vi "Keithley Hangar.vi"() -> ()   [LabVIEW 2013]
uses:
  <vilib>/Platform/TimedLoop/XDataNode/timing_clust.ctl
  <vilib>/Platform/TimedLoop/XDataNode/nitl_modes.ctl
  <vilib>/Platform/TimedLoop/XDataNode/wakeup.ctl
  <vilib>/Instr/_visa.llb/VISA Configure Serial Port (Instr).vi
  <vilib>/Platform/TimedLoop/XDataNode/XDataNode.xnode
  <vilib>/Platform/TimedLoop/XDataNode/XDNodeRunTimeDep.lvlib
panel:
  in  "OK Button":bool
  out "read buffer 3":string
  in  "Unit":string(combo)
  in  "Current":dbl
  in  "CUSTOM COMMAND":string(combo)
  in  "stop":bool
  out "error out":errorcluster
  out "read buffer 2":string
  out "Bytes at Port 3":u32
  in  "RUN Keithley Measurement":bool
  in  "flow control (0:none)":u16(ring) items=["None", "XON/XOFF", "RTS/CTS", "XON/XOFF & RTS/CTS", "DTR/DSR", "XON/XOFF & DTR/DSR"]
  in  "stop bits (10: 1 bit)":u16(ring)=10 items=["1.0"=10, "1.5"=15, "2.0"=20]
  in  "parity (0:none)":enum16{"None", "Odd", "Even", "Mark", "Space"}(ring)
  in  "data bits (8)":u16=8 min=5 max=8 step=1
  in  "baud rate (9600)":u32=9600
  in  "VISA resource name":refnum<visa-resource-name>="COM1"
  in  "Keithley delay (ms)":u32=500
  in  "Set Output Current":bool
  out "actual value":string
  out "Bytes at Port":u32
  out "command to Keithley":string
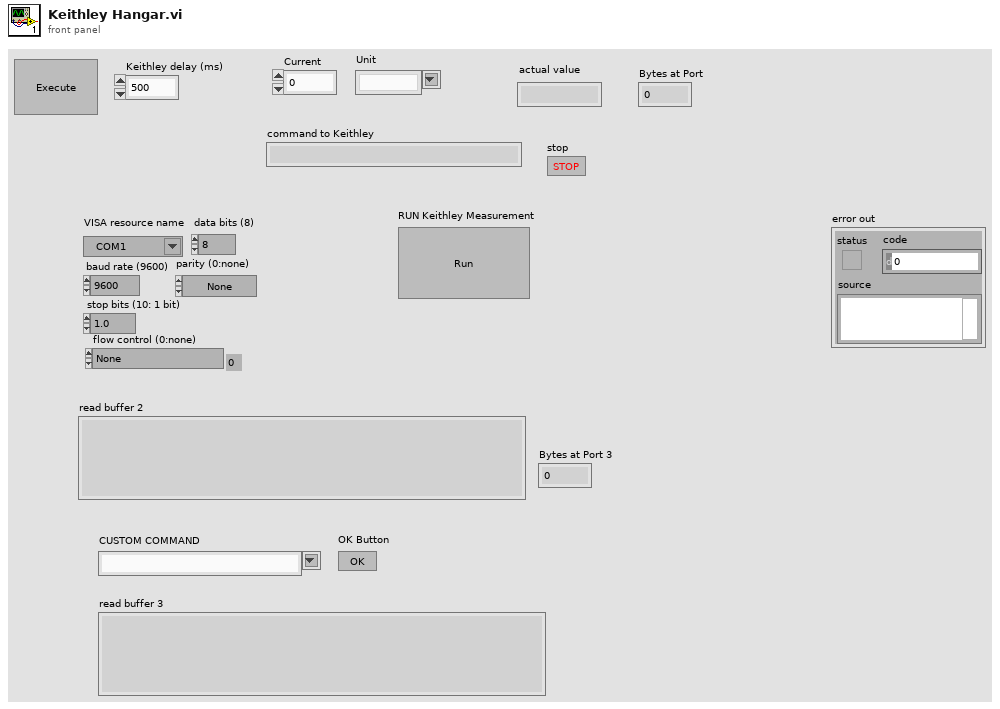
[diagram p1: front panel]
types:
  T1 = typedef "XDNodeRunTimeDep.lvlib/timing_clust.ctl" = cluster{"Expected End [f-1]":u64, "Actual End [f-1]":u64, "Finished Late? [f-1]":bool, "Expected End [i-1]":u64, "Actual End [i-1]":u64, "Finished Late? [i-1]":bool, "Expected Start [i]":u64, "Actual Start [i]":u64, "Expected Start [f]":u64, "Actual Start [f]":u64, "Source Name":string, "Structure Name":string, "Period":i64, "Deadline":i64, "Offset":i64, "Start":i64, "Priority":i32, "Timeout":i32, "Mode":T2, "Wakeup Reason":T3, "Error":errorcluster, "Source Type":string, "Secondary Source Type":string, "Global End Time":u64, "Global Start Time":u64, "Frame Duration":u64, "Iteration Duration":u64, "Assigned CPU":i32, "I/O Scan Engine Mode":u32}
  T2 = typedef "XDNodeRunTimeDep.lvlib/nitl_modes.ctl" = enum32{"No Change", "Process missed periods, maintain original phase", "Discard missed periods, maintain original phase", "Process missed periods, ignore original phase", "Discard missed periods, ignore original phase"}
  T3 = typedef "XDNodeRunTimeDep.lvlib/wakeup.ctl" = enum32{"Normal", "Aborted", "Asynchronous wakeup", "Timing source error", "Timed loop error", "Timeout"}
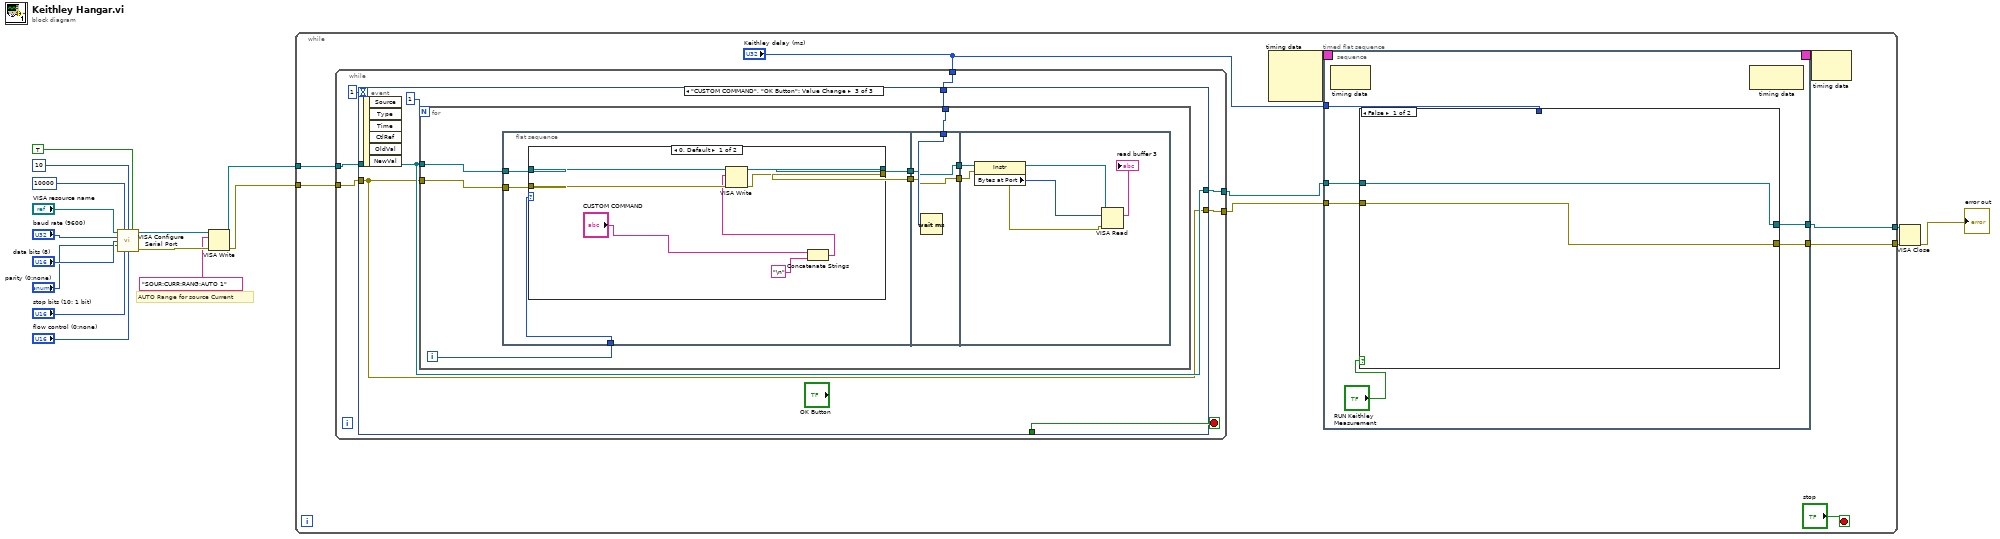
[diagram p0: block diagram]
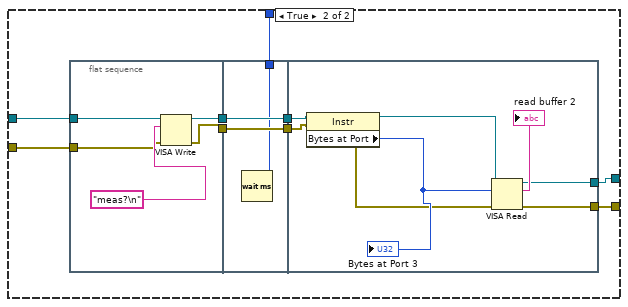
[diagram p2: hidden frame]
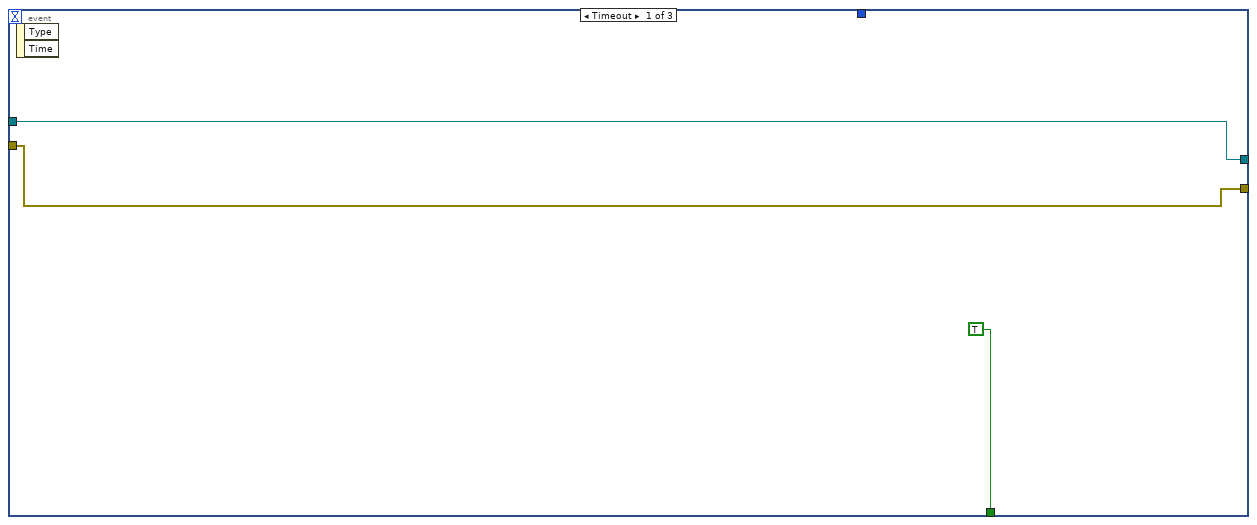
[diagram p3: hidden frame]
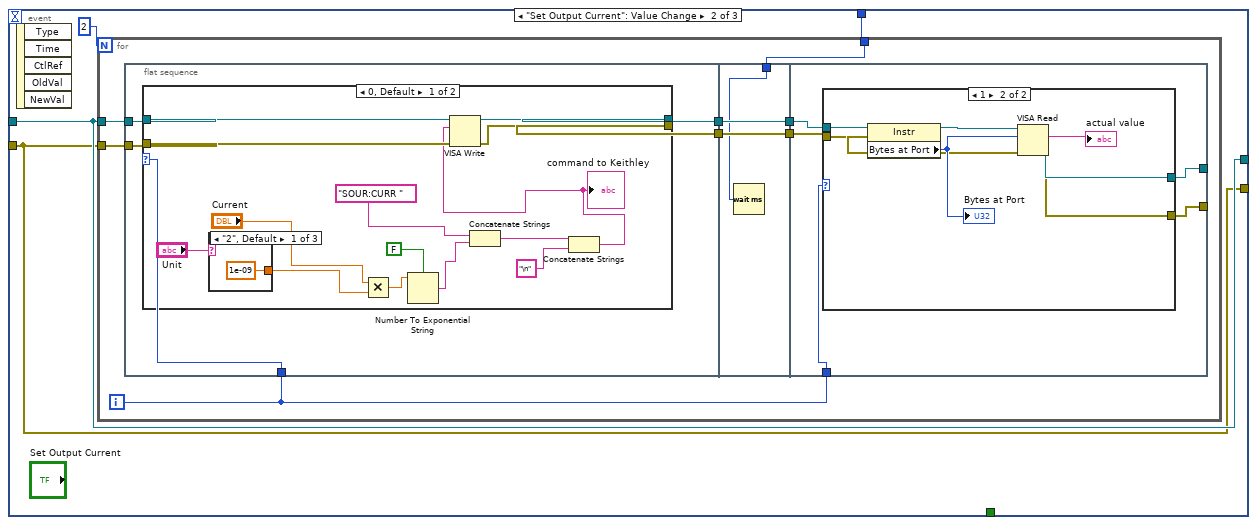
[diagram p4: hidden frame]
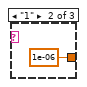
[diagram p5: hidden frame]
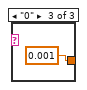
[diagram p6: hidden frame]
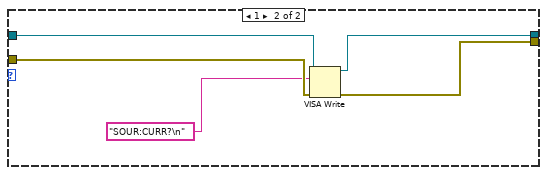
[diagram p7: hidden frame]
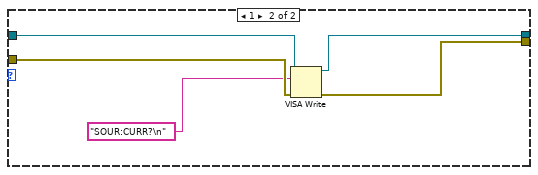
[diagram p9: hidden frame]
diagram:
  # "AUTO Range for source Current"
  n1 = call-poly "VISA Configure Serial Port"("VISA resource name"="VISA resource name", "timeout (10sec)"=u32 10000, "termination char\n(0xA = '\\n' = LF)"=u8 10 ("termination char\n(0xA = '\\n' = LF)"), "Enable Termination\nChar (T)"=TRUE ("Enable Termination\nChar (T)"), "baud rate (9600)"="baud rate (9600)", "data bits (8)"="data bits (8)", "parity (0:none)"="parity (0:none)", "stop bits (10: 1 bit)"="stop bits (10: 1 bit)", "flow control (0:none)"="flow control (0:none)") -> ("VISA resource name out"=w5:refnum<visa-resource-name>, "error out"=w3:errorcluster)  [unwired: 5 in]
  n2 = VISA Write(VISA resource name=w5, write buffer="SOUR:CURR:RANG:AUTO 1", error in (no error)=w3) -> (VISA resource name out=w4:refnum<visa-resource-name>, error out=w2:errorcluster)  [unwired: 1 out]
  n3 = while {
    tunnel: [w25] -> w7
    tunnel: [w24] -> w6
    tunnel: w4 -> [w21]
    tunnel: w2 -> [w20]
    stop <- "stop" stop-if-true
    n4 = while {
      tunnel: "Keithley delay (ms)" -> [w76]
      tunnel: w21 -> [w75]
      tunnel: w20 -> [w74]
      tunnel: [w71] -> w23
      tunnel: [w70] -> w22
      stop <- w72 stop-if-true
      n5 = event shown="[2] \"CUSTOM COMMAND\", \"OK Button\": Value Change" {
        selector: _ -> [_ _ _]
        dyn-events: _ -> [_ _ _]
        timeout: 1 -> [_ _ _]
        tunnel: w76 -> [_ w82 w139]
        tunnel: w75 -> [w78 w81 w138]
        tunnel: w74 -> [w77 w80 w137]
        tunnel: [TRUE _ _] -> w72
        tunnel: [w78 w81 w138] -> w71
        tunnel: [w77 w80 w137] -> w70
        event Timeout {
          n6 = event-data() -> ()  [unwired: 1 in, 2 out]
        }
        event "Set Output Current": Value Change {
          n7 = event-data() -> ()  [unwired: 1 in, 5 out]
          n8 = for {
            N: 2 -> [_]
            tunnel: w82 -> [w86]
            tunnel: w81 -> [w85]
            tunnel: w80 -> [w84]
            i -> [w89]
            n9 = flat-sequence {
              tunnel: [w96] -> w91
              tunnel: w89 -> [w95]
              tunnel: [w94] -> w88
              tunnel: w85 -> [w93]
              tunnel: w84 -> [w92]
              tunnel: w91 -> [w121]
              tunnel: [w121] -> w90
              tunnel: w88 -> [w120]
              tunnel: [w120] -> w87
              tunnel: w86 -> [w119]
              tunnel: w90 -> [w126]
              tunnel: w89 -> [w125]
              tunnel: w87 -> [w124]
              tunnel: [w123] -> _
              tunnel: [w122] -> _
              frame #0 {
                n10 = case shown="0, Default" w95 {
                  tunnel: [w110 w115] -> w96
                  tunnel: [w109 w114] -> w94
                  tunnel: w93 -> [w108 w117]
                  tunnel: w92 -> [w107 w118]
                  frame 0, Default {
                    n11 = case shown="\"2\", Default" "Unit" {
                      tunnel: [1e-09 ("y") 1e-06 ("y") 0.001 ("y")] -> w97
                      frame "2", Default {
                      }
                      frame "1" {
                      }
                      frame "0" {
                      }
                    }
                    n12 = Multiply(x="Current", y=w97) -> (x*y=w100:dbl)
                    n13 = Number To Exponential String(number=w100, 1:FALSE ("use system decimal point (T)")) -> (E-format string=w105:string)  [unwired: 2 in]
                    n14 = Concatenate Strings("SOUR:CURR " ("string"), w105) -> (w103:string)
                    n15 = Concatenate Strings(w103, "\n" ("string")) -> (w102:string)
                    "command to Keithley" <- w102
                    n16 = VISA Write(VISA resource name=w108, write buffer=w102, error in (no error)=w107) -> (VISA resource name out=w110:refnum<visa-resource-name>, error out=w109:errorcluster)  [unwired: 1 out]
                  }
                  frame 1 {
                    n17 = VISA Write(VISA resource name=w117, write buffer="SOUR:CURR?\n" ("string"), error in (no error)=w118) -> (VISA resource name out=w115:refnum<visa-resource-name>, error out=w114:errorcluster)  [unwired: 1 out]
                  }
                }
              }
              frame #1 {
                n18 = Wait (ms)(milliseconds to wait=w119) -> ()  [unwired: 1 out]
              }
              frame #2 {
                n19 = case shown="1" w125 {
                  tunnel: w126 -> [w128 w132]
                  tunnel: w124 -> [w127 w131]
                  tunnel: [w128 w130] -> w123
                  tunnel: [w127 w129] -> w122
                  frame 0, Default {
                  }
                  frame 1 {
                    n20 = property class="Instr"(reference=w132, error in=w131) -> (reference out=w134:refnum<visa-resource-name>, error out=w133:errorcluster, "Bytes at Port"=w136:u32)
                    "Bytes at Port" <- w136
                    n21 = VISA Read(VISA resource name=w134, byte count=w136, error in (no error)=w133) -> (VISA resource name out=w130:refnum<visa-resource-name>, read buffer=→"actual value":string, error out=w129:errorcluster)  [unwired: 1 out]
                  }
                }
              }
            }
          }
        }
        event "CUSTOM COMMAND", "OK Button": Value Change {
          n22 = event-data() -> ()  [unwired: 1 in, 6 out]
          n23 = for {
            N: 1 -> [_]
            tunnel: w139 -> [w145]
            tunnel: w138 -> [w144]
            tunnel: w137 -> [w143]
            i -> [w147]
            n24 = flat-sequence {
              tunnel: [w153] -> w148
              tunnel: w147 -> [w152]
              tunnel: [w151] -> w146
              tunnel: w144 -> [w150]
              tunnel: w143 -> [w149]
              tunnel: w148 -> [w167]
              tunnel: w146 -> [w166]
              tunnel: w145 -> [w168]
              tunnel: [w167] -> w142
              tunnel: [w166] -> w141
              tunnel: w142 -> [w171]
              tunnel: w141 -> [w170]
              frame #0 {
                n25 = case shown="0, Default" w152 {
                  tunnel: [w160 w162] -> w153
                  tunnel: [w159 w161] -> w151
                  tunnel: w150 -> [w158 w164]
                  tunnel: w149 -> [w157 w165]
                  frame 0, Default {
                    n26 = Concatenate Strings("CUSTOM COMMAND", "\n" ("string")) -> (w155:string)
                    n27 = VISA Write(VISA resource name=w158, write buffer=w155, error in (no error)=w157) -> (VISA resource name out=w160:refnum<visa-resource-name>, error out=w159:errorcluster)  [unwired: 1 out]
                  }
                  frame 1 {
                    n28 = VISA Write(VISA resource name=w164, write buffer="SOUR:CURR?\n" ("string"), error in (no error)=w165) -> (VISA resource name out=w162:refnum<visa-resource-name>, error out=w161:errorcluster)  [unwired: 1 out]
                  }
                }
              }
              frame #1 {
                n29 = Wait (ms)(milliseconds to wait=w168) -> ()  [unwired: 1 out]
              }
              frame #2 {
                n30 = property class="Instr"(reference=w171, error in=w170) -> (reference out=w172:refnum<visa-resource-name>, error out=w169:errorcluster, "Bytes at Port"=w174:u32)
                n31 = VISA Read(VISA resource name=w172, byte count=w174, error in (no error)=w169) -> (read buffer=→"read buffer 3":string)  [unwired: 3 out]
              }
            }
          }
        }
      }
    }
    n32 = node-c288() -> (w27:T1)  [unwired: 3 in]
    n33 = timed-sequence {
      timing: w27 -> [_]
      timing-out: [_] -> w26
      tunnel: [w32] -> w25
      tunnel: [w31] -> w24
      tunnel: "Keithley delay (ms)" -> [w30]
      tunnel: w23 -> [w29]
      tunnel: w22 -> [w28]
      n34 = timed-flat-sequence {
        tunnel: [w37] -> w32
        tunnel: [w36] -> w31
        tunnel: w30 -> [w35]
        tunnel: w29 -> [w34]
        tunnel: w28 -> [w33]
        n35 = node-c288() -> ()  [unwired: 1 in, 1 out]
        n36 = case shown="False" "RUN Keithley Measurement" {
          tunnel: w35 -> [_ w45]
          tunnel: [w40 w44] -> w37
          tunnel: [w39 w43] -> w36
          tunnel: w34 -> [w40 w42]
          tunnel: w33 -> [w39 w41]
          frame False {
          }
          frame True {
            n37 = flat-sequence {
              tunnel: [w54] -> w49
              tunnel: [w53] -> w48
              tunnel: w42 -> [w51]
              tunnel: w41 -> [w50]
              tunnel: w49 -> [w57]
              tunnel: [w57] -> w47
              tunnel: w48 -> [w56]
              tunnel: [w56] -> w46
              tunnel: w45 -> [w55]
              tunnel: w47 -> [w61]
              tunnel: w46 -> [w60]
              tunnel: [w59] -> w43
              tunnel: [w58] -> w44
              frame #0 {
                n38 = VISA Write(VISA resource name=w51, write buffer="meas?\n" ("write buffer 2"), error in (no error)=w50) -> (VISA resource name out=w54:refnum<visa-resource-name>, error out=w53:errorcluster)  [unwired: 1 out]
              }
              frame #1 {
                n39 = Wait (ms)(milliseconds to wait=w55) -> ()  [unwired: 1 out]
              }
              frame #2 {
                n40 = property class="Instr"(reference=w61, error in=w60) -> (reference out=w63:refnum<visa-resource-name>, error out=w62:errorcluster, "Bytes at Port"=w65:u32)
                "Bytes at Port 3" <- w65
                n41 = VISA Read(VISA resource name=w63, byte count=w65, error in (no error)=w62) -> (VISA resource name out=w58:refnum<visa-resource-name>, read buffer=→"read buffer 2":string, error out=w59:errorcluster)  [unwired: 1 out]
              }
            }
          }
        }
        n42 = node-c288() -> ()  [unwired: 1 in, 1 out]
      }
    }
    n43 = node-c288(w26) -> ()  [unwired: 1 out]
  }
  n44 = VISA Close(VISA resource name=w7, error in (no error)=w6) -> (error out=→"error out":errorcluster)
